vi "Main.vi"() -> ()   [LabVIEW 2013]
uses:
  Controls/Setup - Part Details - Item Details.ctl
  Controls/Combo Box.ctl
  Controls/Execute - Info.ctl
  Controls/Enum - SRTRS State.ctl
  Controls/DB - Refnums.ctl
  Controls/Report Files Cluster.ctl
  Controls/DB - Refnums II.ctl
  Controls/Transaction Cluster.ctl
  Controls/Report List Cluster.ctl
  Controls/DB - Logon Info.ctl
  Controls/DB - Logon Extra Info.ctl
  Controls/ET3500 Program Status.ctl
  <vilib>/Utility/miscctls.llb/LVRowAndColumnUnsignedTypeDef.ctl
  <vilib>/Utility/miscctls.llb/LVPointTypeDef.ctl
  Controls/Execute - Color Init.ctl
  <vilib>/Utility/miscctls.llb/LVRowAndColumnTypeDef.ctl
  Controls/Enum - Tabs.ctl
  Controls/DB - Setup Item Enum.ctl
  Controls/Msgbox Timer Cluster.ctl
  Controls/cRIO RW Enum.ctl
  Controls/DB - Execute Transaction Enum.ctl
  Controls/DB - [TransactionResult] Enum.ctl
  Controls/DB - CMS Execute Active Process.ctl
  Controls/DB - [Execute].[ActiveProcess] Enum.ctl
  Controls/DB - Execute ReportList Enum.ctl
  Controls/DB - [TransactionNo],[OrderNo].ctl
  Controls/DB - Master Data OutputSet SQL.ctl
  Controls/DB - OpenClose.ctl
  Controls/Report Additional Details Cluster.ctl
  Controls/Message Code - Enum.ctl
  <vilib>/event_ctls.llb/eventvkey.ctl
  Controls/DB - Master Data Material Enum.ctl
  Controls/DB - Master Data Procedure Enum.ctl
  <vilib>/Utility/miscctls.llb/LVSelectionTypeDef.ctl
  Controls/DB - [Config].[Parameters].[ParameterId] Values.ctl
  Controls/DB - [Config].[GeneralSetting].[SystemId] Values.ctl
  Controls/Key Enum.ctl
  Controls/Global SRTRS.vi
  <vilib>/Utility/config.llb/Write Key (String).vi
  <vilib>/nisyscfg/Close (System).vi
  <vilib>/addons/database/Connection.llb/DB Tools Open Connec (String).vi
  <vilib>/Utility/config.llb/Write Key (Boolean).vi
  <vilib>/express/express shared/transition.llb/Dynamic To Waveform Array.vi
  <vilib>/express/express signal manip/GetorSetDDTAttributes/Set DDT Attributes/SetT0.vi
  <vilib>/express/express shared/transition.llb/Waveform Array To Dynamic.vi
  <vilib>/Waveform/WDTOps.llb/WDT Get Waveform Subset DBL.vi
  <vilib>/express/express signal manip/GetorSetDDTAttributes/Set DDT Attributes/Set DDT Properties.xnode
  <vilib>/Utility/config.llb/NI_LVConfig.lvlib
  <vilib>/nisyscfg/nisyscfg.lvlib
  <vilib>/FTP/NI_FTP.lvlib
  <vilib>/addons/database/NI_Database_API.lvlib
  SubVIs/tool_Unicode_Convert ASCII to Unicode (Scalar).vi
panel:
  out "[Remarks] +[ShortDescription] Debug":string caption="[Remarks] +[ShortDescription]"
  out "Time To Log Off":dbl(slide)=599.8004469871521 scale=0.0..600.0
  in  "Tab Header":enum32{"Header"}(tab)
  out "Plant and Furnace Name":string="One Subsea Johor, SRSB-A1, Administrator"
  in  "Close":bool
  out "ApplicationName":string caption="[LogoName]"
  out "LogoName":picture
  in  "Debug Close":bool
  in  "Setup Load Debug":bool
  in  "Tab Footer":enum32{"Footer"}(tab)
  out "date/time string":string="Nov 22, 2014  15:42:28"
  out "[Remarks] +[ShortDescription]":string
  in  "Tab Body":T1(tab)
  in  "Search Setup":bool caption="Setup Save"
  in  "Setup New":bool
  in  "Setup Edit":bool=TRUE
  out "Transaction No":string caption="Transaction No."
  in  "Tab Setup":enum32{"Part Details", "Furnace Settings"}(tab) caption="Setup"
  in  "SAPMaterial Description (Long) Setup Tab":bool
  in  "SAPProduction Long Text":bool
  in  "Channel Mapping":T2 caption="Channels Mapping"
  in  "Item Details":T3={"Order No."="", "Oper. No."="", "Qty."=1, "NCR No."="", "NCR Boolean"=FALSE, "Customer No."="", "Customer Name"="", "Project"="", "Sales Order"="", "Item No."="", "Material"="", "Revision"="", "Material Description"="", "Serial No."="", "UnitOfQty"=""} {"Qty." min=1 max=99}
  in  "Part Details Delete":bool
  in  "Part Details Add":bool
  in  "Notes":string
  in  "No.":i32=1 caption="Item Number" min=1 max=100
  out "Setup Thermocouple Location":picture caption="Thermocouples Position: Outline"
  in  "Part Details":i32(listbox)=-1
  in  "Plot":T4
  in  "FHS Ramp Rate Units":string="°C"
  in  "Ramp Rate (Brackets)":string caption="(       / Hour )"
  in  "Target Temperature (Brackets)":string caption="(        )"
  in  "Hold Time (Brackets)":string caption="(HH:MM)"
  in  "Results Output":cluster{"Output Set":T5, "Description":string}={"Output Set"="001", "Description"="Output Set 1"}
  in  "Extra Rev":string caption="Rev."
  in  "Extra WPS":string caption="WPS"
  in  "Read ET3500 Program":bool
  in  "FHS Target Temp Units":string="°C"
  in  "MCListBox AWPS Remove Button":bool
  in  "MCListBox AWPS Add Button":bool
  out "Equipment Details":i32(listbox)=-1
  out "Furnace Details":T6={"Furnace Serial No"="A1234A1", "Last Calibration Date"="2012-11-22", "Next Calibration Due Date"="2014-11-22"}
  in  "Additional WPS/Ref":T7 caption="Additional WPS"
  in  "WPS Details Setup":T8={"WPS/Ref"="", "Rev"="", "Hold Temperature"="", "WPS Details Temperature Units"="°C", "Hold Time (HH:MM)"="", "Inactive"=FALSE} caption="WPS Details"
  in  "MCListBox AWPS":i32(listbox)=-1 caption="Additional WPS/Ref MCListBox"
  in  "MCListBox FHS Setup Add Button":bool
  in  "MCListBox FHS Setup Remove Button":bool
  in  "MCListBox FHS Setup":i32(listbox)=-1 caption="Furnace Heating Sequence"
  in  "Setup Save":bool
  out "TransactionRunNo":string caption="Run No."
  in  "Copy New":bool caption="Setup Save"
  in  "Transaction Details":bool
  in  "System Status [CaptionOnly] 2":string caption="System Status"
  in  "Process Status [CaptionOnly]":string caption="Process Status"
  out "% Hold. Time Completed (Num)":i32 format="%d%%"
  out "Overall Status":bool
  out "Sequence Status":string caption="Sequence"
  in  "Parameter":bool
  out "ET3504 Status":string="Program [33]. Segment [End].Program Status [Not Running]. ET3500 Simulate Mode." caption="Furnance"
  out "Info.":T9={"Ref WPS"="", "Hold. Temp."="", "Info. Temperature Units"="°C", "Variant Allowed (Hold Temp)"=5.0, "Info. Temperature Units 2"="°C", "Variant Allowed (Hold Temp)"=FALSE, "Hold. Time (hour:minute)"="", "Variant Allowed (Hold Time)"=30.0, "Variant Allowed (Hold Time)"=FALSE, "WPS"=""} {"Variant Allowed (Hold Temp)" format="%.1f"}
  out "Hold Time Completed":bool
  out "Process Completed":bool
  out "% Hold. Time Completed":dbl(slide) scale=0.0..100.0
  out "Transaction No (Execute)":string caption="Transaction No."
  out "Key Values":T10={"Recording Duration"=0.0, "Remaining Hold Time"=0.0, "Current Temp"=25.108964136983314, "Key Values Temperature Units"="°C"} {"Current Temp" format="%#_4f"; "Remaining Hold Time" format="%<%H:%M>t"; "Recording Duration" format="%<%H:%M:%S>t"}
  out "Chart":dynamicdata(graph)
  in  "Recipe Start":bool
  in  "Recipe Stop":bool
  out "cRIO Status":string="DAQ Waiting to Start. cRIO Simulate Mode." caption="Data Logger"
  out "TransactionRunNo (Execute)":string caption="Run No."
  in  "Probe Number [CaptionOnly]":string caption="Probe Number"
  in  "Create Report [CaptionOnly]":string caption="Create Report"
  in  "Retrieve Raw Data [CaptionOnly]":string caption="Retrieve Raw Data"
  in  "Display Report [CaptionOnly]":string caption="Display Report"
  in  "cRIO FTP Copy":bool caption="Report Execute Search"
  in  "FTP File List":i32(listbox)=-1
  in  "cRIO  Search":bool caption="Report Execute Search"
  in  "FTP Month":i16=11 caption="Month" min=1 max=12 format="%02d"
  in  "FTP Year":i16=2014 caption="Year" min=2013 max=2099
  in  "Report Open":bool caption="Report Execute Search"
  in  "Report List":i32(listbox)=-1 caption="List"
  in  "Report Generate":bool
  in  "Raw Data File (Report Tab)":path caption="Raw Data File"
  in  "Report Selection":T11={"Date Start"=timestamp(3498882134.864412 s since 1904-01-01), "Date End"=timestamp(3499486934.864412 s since 1904-01-01), "Selection Transaction No"="", "Selection Order No"="", "Report Execute Search "=FALSE} caption="Selection" {"Date End" format="%<%Y/%m/%d>T"; "Date Start" format="%<%Y/%m/%d>T"}
  in  "Master Data Tab":enum32{"Material", "WPS", "Layout"}(tab) caption="Tab Master Data"
  in  "Material Reference [CaptionOnly]":string caption="Reference"
  in  "Master Data Ref Material":string(combo) caption="Material"
  in  "Material Details [CaptionOnly]":string caption="Material Details"
  in  "SAPMaterial Description (Long) Master Data Tab":bool
  in  "Material Paste":bool caption="Material Browse"
  in  "Material Copy":bool caption="Material Browse"
  in  "Material":T12 caption="Header"
  in  "Material New":bool
  in  "Material Browse":bool
  in  "Material Save":bool caption="Material Add"
  out "Master Data Thermocouple Location":picture caption="Thermocouples Position: Outline"
  in  "WPS Details [CaptionOnly]":string caption="WPS Details"
  in  "MasterData FHS Target Temp Units":string="°C"
  in  "MasterData FHS Ramp Rate Temp Units":string="°C"
  in  "WPS Details Master Data":T13={"Master Data WPS/Ref"="", "Master Data Rev"="", "Master Data Hold Temperature"="", "Master Data Temperature Units"="°C", "Master Data Hold Time (HH:MM)"="", "Inactive"=FALSE} caption="Header"
  in  "MCListBox FHS Master Data":i32(listbox)=-1 caption="Furnance Heating Sequence"
  in  "Master Data New":bool
  in  "Master Data Save":bool
  in  "MCListBox FHS Master Data Remove Button":bool
  in  "MCListBox FHS Master Data Add Button":bool
  in  "Output Details [CaptionOnly]":string caption="Output Details"
  in  "Admin (User/Equipment) Tab":enum32{"User", "Equipment"}(tab)
  in  "User Details [CaptionOnly]":string caption="User Details"
  in  "Equipment Details [CaptionOnly]":string caption="Equipment Details"
  in  "System Status [CaptionOnly]":string caption="System Status"
  out "Material Image File":errorcluster
  out "Statistics":errorcluster
  out "Chart":errorcluster
  out "Property Node Error":errorcluster
  in  "Mytab":T14(tab)
  in  "MasterData\\Language":path=path "c:/temp/SRTRS4070/MasterData/Language"
  in  "MasterData\\Layout":path=path "c:/temp/SRTRS4070/MasterData/Layout"
  in  "Setup":path=path "c:/temp/SRTRS4070/Setup"
  in  "MasterData\\WPS":path=path "c:/temp/SRTRS4070/MasterData/WPS" caption="Master Data WPS"
  in  "MasterData\\JPG":path=path "c:/temp/SRTRS4070/MasterData/JPG"
  in  "Data":path=path "c:/temp/SRTRS4070/Data" caption="Folder Data"
  in  "Excel":path=path "c:/temp/SRTRS4070/Excel" caption="Folder Excel"
  in  "Logs":path=path "c:/temp/SRTRS4070/Logs"
  in  "Reports":path=path "c:/temp/SRTRS4070/Reports" caption="Folder Report"
  in  "Temp_Host":path=path "c:/temp/SRTRS4070_Host/Temp_Host"
  in  "Data_Host":path=path "c:/temp/SRTRS4070_Host/Data_Host" caption="Folder Data"
  in  "Logs_Host":path=path "c:/temp/SRTRS4070_Host/Logs_Host"
  in  "Dummy Load":bool caption="Show Debug Tab"
  out "Update English Captions":bool
  out "Display Reference Chart":bool=TRUE
  out "Settings Load Sequence":i32[](array[numeric])=[0, 1, 2]
  out "Date Format (UserDefined)":string="%Y-%m-%d"
  out "Starting Number for Transaction number":i32=1000000001
  out "Display Start Stop Marker":bool=TRUE
  out "ini File Error":errorcluster
  out "Log Off Timer (s)":i32=600
  out "Chart Separation by Order#":bool=TRUE
  out "Lite Version":bool
  out "stp file Error Out":errorcluster
  out "Furnace Number":string="03"
  out "Running Number":i32=829
  out "Show Debug TAB":bool=TRUE caption="Show Debug Tab"
  out "Show LabVIEW Error":bool
  out "Application:Name":string="LabVIEW.exe"
  out "Metrics:Code Size":u32=1762288 format="%#.3p"
  out "MCListBox Ref":refnum<vi>[](array[refnum])
  in  "CellBG ColHdrs":u32(colorbox)=11776947
  in  "CellBG Unused Cells":u32(colorbox)=16777238
  in  "CellBG New Cells":u32(colorbox)=16777225
  out "Latest stp file":path=path "c:/temp/SRTRS4070/Setup/2014/11/0090300828_20141120_120827.stp"
  out "LabVIEW Directory Path":path=path "C:/Program Files (x86)/National Instruments/LabVIEW 2013"
  out "All Calibration Date Valid":bool
  out "Calibration Date OK":bool[](array[boolean])
  out "User":string="admin"
  in  "Edit WPS in Setup":bool
  out "Final Logoff Timer (s)":i32=600
  out "Temperature Units":refnum<vi>[](array[refnum])
  out "SRTRS4070 Host Folder":string="c:\\temp\\SRTRS4070_Host"
  out "SRTRS4070 Folder (Server Folder)":string="c:\\temp\\SRTRS4070"
  out "LogoName":errorcluster
  out "Current VI's path":path=path "C:/Users/CK/workspace/LabVIEW/Stress Relief Temperature Recording/VIs/Main.vi"
  out "Application Directory":path=path "C:/Users/CK/workspace/LabVIEW/Stress Relief Temperature Recording"
  out "[TimeZone]":string="+8"
  out "Enable Central Monitoring":bool=TRUE
  out "File Version":string="ver. 13.0f1"
  out "Plant and Furnace Name (B4 Logon)":string="ver. 13" caption="Plant and Furnace Name"
  out "[LogoFile]":string="C:\\Temp\\SRTRS4070_Host\\Temp_Host\\OneSubseaLogo.jpg"
  out "Caption Error Out":errorcluster
  out "Enable AMS Update":bool=TRUE
  out "Equipment ID Notice Due List":string
  out "Equipment Details Complete":bool caption="Output Set Complete"
  in  "Setup New Toggle":bool caption="Report Generate Procedure"
  in  "Search [OrderNo] Toggle":bool caption="Report Generate Procedure"
  out "From Search Button":bool caption="Report Generate Procedure"
  out "Channel to Probe Mapping":cluster{"Channel to Probe Mapping":string}={"Channel to Probe Mapping"="1,2,3,4,5,6,7,8,9,10,11,12,13,14,15,16"}
  out "Probe List":i32[](array[numeric])
  out "Probe List Valid":bool
  out "cRIO Channel List":i32[](array[numeric])
  out "Empty String in Mandatory Field":bool
  out "WPS Details Complete":bool
  out "FHS Last Row":i32
  out "[Setup].[Item] COLUMN_NAME":string[](array[string])=["TransactionNo", "ItemNo", "OrderNo", "OperationNo", "Qty", "UnitOfQty", "NCRIndicator", "NCRNo", "CustomerID", "Customer", "Project", "SalesOrderNo", "SalesOrderItemNo", "MaterialNo", "MaterialDesc", "MaterialRev", "SerialNos", "Notes", "TC01", "TC02", "TC03", "TC04", "TC05", "TC06", "TC07", "TC08", "TC09", "TC10", "TC01Plot", "TC02Plot", "TC03Plot", "TC04Plot", "TC05Plot", "TC06Plot", "TC07Plot", "TC08Plot", "TC09Plot", "TC10Plot", "Inactive"]
  out "[Setup].[Item] DATA_TYPE":string[](array[string])=["int", "int", "nvarchar", "nvarchar", "int", "nvarchar", "nvarchar", "nvarchar", "nvarchar", "nvarchar", "nvarchar", "nvarchar", "nvarchar", "nvarchar", "nvarchar", "nvarchar", "nvarchar", "nvarchar", "nvarchar", "nvarchar", "nvarchar", "nvarchar", "nvarchar", "nvarchar", "nvarchar", "nvarchar", "nvarchar", "nvarchar", "nvarchar", "nvarchar", "nvarchar", "nvarchar", "nvarchar", "nvarchar", "nvarchar", "nvarchar", "nvarchar", "nvarchar", "bit"]
  out "[Setup].[Item] PRECISION":string[](array[string])=["10", "10", "10", "5", "10", "5", "50", "20", "10", "30", "30", "10", "6", "20", "60", "3", "255", "255", "2", "2", "2", "2", "2", "2", "2", "2", "2", "2", "1", "1", "1", "1", "1", "1", "1", "1", "1", "1", "1"]
  out "[IsMandatory]":string[](array[string])=["0", "0", "0", "0", "-1", "0", "-1", "0", "0", "-1", "", "", "0", "0"]
  out "[IsMandatory]\nLabel.Text":string[](array[string])=["Customer No.", "Project", "Material"]
  in  "Search Setup Toggle":bool caption="Report Generate Procedure"
  out "Revision Toggle":string caption="Report Generate Procedure"
  out "Part Details Complete":bool caption="WPS Details Complete"
  out "Output Set Details Complete":bool caption="Output Set Complete"
  out "FHS Hold Details Complete":bool caption="WPS Details Complete"
  out "Equipment ID Due List":string
  out "TCxxPlots 2":string[][](array[string])
  out "TCxxPlots":bool
  out "<current hold time> ON Failing Hold Time Variance":string
  in  "Simulate Hold Time Inc (s)":dbl=2400.0
  out "Toggle ET3500 Error":string
  in  "Simulate Hold Temp Inc":dbl=20.0
  out "Final Target Temperature":cluster{"Final Target Temperature":string}
  in  "Parameter Buffer":T15
  out "Parameter (End Dwell Time)":timestamp
  out "Parameter (Start Dwell Time)":timestamp
  out "ET3500 Error":errorcluster
  in  "Simulate ET3500":bool=TRUE
  out "Parameter Cluster (Scaled)":T16={"ProgramNumber"=1, "CurProg"=33, "CurSeg"=1, "ProgStatus"=1, "ProgTimeLeft (min)"=0.0, "PVIn (DegC)"=25.108964136983314, "SPIn (s)"=0.0, "SegTimeLeft (min)"=9.0}
  in  "Simulate ET3500 Error":bool
  in  "Final Target Temp Offset":i32
  in  "Stop On Final Target Temperature":bool=TRUE
  out "Final Target + Offset\n(Updated Only when active)":i32
  out "Seq-Seg Info":T17
  out "Uploaded to ET":bool caption="ET Program Downloaded"
  in  "Simulate Hold Temp Inc":bool
  in  "Simulate Hold Time Inc":bool
  out "Hold Time %":string
  out "<current temperature> ON Failing Hold Temp Variance":string
  out "cRIO Time Sync Schedule":i32=700 caption="cRIO Time Sync Tolerance"
  in  "Simulate cRIO No Data":bool
  out "cRIO DAQ Started":bool
  out "cRIO Error":errorcluster
  out "cRIO Cycle Count":i32
  out "cRIO shared variable RT Library":string="ni.var.psp://192.168.1.50/RT Library"
  out "VISA resource name RS232":string="visa://192.168.1.50/ASRL1::INSTR"
  out "Samples/ch Count":i32
  out "cRIO COM Port":string="visa://192.168.1.50/ASRL1::INSTR"
  out "Host COM Port":string="COM3"
  out "cRIO IP":string="192.168.1.50"
  out "cRIO Folder":string="/c/ni-rt/LabVIEW Data/SRTRS4070"
  in  "Simulate cRIO":bool=TRUE caption="Simulate cRIO Data"
  in  "Use Host COM Port":bool
  out "cRIO Data Retention":i32=3
  out "cRIO Timestamp":timestamp
  in  "Simulate cRIO Comm Error":bool
  in  "Simulate cRIO Started":bool
  out "1st TC":dbl
  out "Data Path Name (cRIO SV)":string
  out "Files in cRIO":string[](array[string])
  out "cRIO File IO Status (updated at File creation only)":bool[](array[boolean])
  out "Check DAQ Started Loop Count":i32
  out "Day cRIO Time is SET":string
  out "SV and ini Data File Name Match. (Recovery)":bool
  out "Simulated TimeStamp":timestamp
  out "cRIO Time Sync Tolerance":i32=60
  out "Source File Path (on RT Target)":string
  out "Destination Folder (on Local Host)":path
  out "Destination File Path (on local host)":path
  out "cRIO FTP Module (Error Out)":errorcluster
  out "Data File Error":errorcluster
  out "Logged File Ref":refnum<file>
  out "Time to next sample (s)":dbl
  out "Host Sampling Interval (s)":dbl=1.0
  in  "Time Target (s)":dbl format="%#_13g"
  out "Raw Data File":string
  out "[StartRecordTime]":string
  out "RecoveryFlag":bool
  out "Recovered Data Size":i32[](array[numeric])
  out "Calculate Parameters from raw Data":string[](array[string])
  out "Variant Allowed (Hold Time) (raw Data)":bool
  out "Variant Allowed (Hold Temp) (raw Data)":bool
  out "|Max - Hold Temp|":dbl
  out "|Min - Hold Temp|":dbl
  out "|Hold - Hold Time|":dbl
  in  "Sort Order":bool caption="Include MetaData"
  in  "Include MetaData":bool=TRUE
  out "ReportList Cluster":T18
  out "Transaction (Report Buffer)":T19
  out "List Of Files From Selected Reports":string[](array[string])
  out "YYYYmm":string
  out "Details From .stp and Parameters":string[](array[string])
  out "Order No":string[](array[string])
  in  "Report.Create.PDF":bool=TRUE caption="Create PDF file at end of Recipe"
  in  "Report.Create.Excel":bool=TRUE caption="Create EXCEL file at end of Recipe"
  out "No Of Orders":i32
  out "Report Files Cluster":T20
  in  "Report Generate Toggle":bool=TRUE caption="Report Generate Procedure"
  out "Logon (Report Buffer)":T21
  out "Msgbox":errorcluster
  out "Ascending":bool
  out "Template File":path
  out "Layout ID":string
  out "Manual Stop":bool caption="Manual Stop Flag"
  out "Stop Log off Event Structure":bool=TRUE
  in  "------------------------------------        Setup TAB      ------------------------------------":string caption="------------------------------------        Setup Tab     ------------------------------------"
  in  "---------------------------------       Master Data (Material)      -----------------------------":string
  out "Temp Array":string[](array[string])
  out "Time has Elapsed":bool
  out "Quit Flag":bool=TRUE
  out "Recipe Start Flag":bool
  out "Recipe Stop Flag":bool
  out "WPS Details Master Data: Mouse Down":u32 caption="Time"
  out "Process t0":timestamp
  out "MasterData Image File Path":path caption="MasterDate Image File Path"
  in  "------------------------------------        Master Data       -----------------------------------":string
  in  "------------------------------------        MCListBox       ------------------------------------":string
  in  "-------------------------------             Report TAB        ------------------------------------":string caption="------------------------------------             Report          ------------------------------------"
  in  "------------------------------------        Part Details       ------------------------------------":string
  out "StateMachine for Main Process":T22=enum."QUIT" caption="Enum"
  out "Show Scrollbars":bool=TRUE
  out "WPS Details Master Data: Value Change":u32
  out "% Hold Flashing FLAG":bool caption="Time has Elapsed"
  in  "Master Data Delete":bool
  in  "Material Delete":bool
  in  "------------------------------------        Execute TAB      ------------------------------------":string caption="------------------------------------        Setup Tab     ------------------------------------"
  in  "------------------------------------        Simulate TAB      ------------------------------------":string caption="------------------------------------        Setup Tab     ------------------------------------"
  in  "Copy Setup":bool caption="Setup Save"
  in  "Paste Setup":bool caption="Setup Save"
  in  "cRIO Set Time":bool
  out "No. of Items":i32
  in  "Reset Log off Display Timer":bool caption="Reset"
  out "MHandler":errorcluster caption="Message Handler Error"
  in  "DB - Active Process":bool=TRUE
  in  "DB - Message":bool=TRUE
  in  "DB - Report":bool=TRUE
  in  "DB - Logon":bool=TRUE
  in  "DB - Transaction":bool=TRUE
  in  "DB - Setup Item (Part Details)":bool=TRUE
  in  "DB - Master Data Load":bool=TRUE
  in  "DB - Master Data Save":bool=TRUE
  out "DB":errorcluster
  out "DB Refnums":T23
  out "[Config].[Parameter]":string[][](array[string])=[["AllowWpsEdit", "0"], ["ChartSeparation", "1"], ["DataLogInterval", "1"], ["DateFormat", "%Y-%m-%d"], ["DisplayRefChart", "1"], ["EnableCmsUpdate", "1"], ["NotifySeverity", "5,6,8,9"], ["PermittedTempDiff", "5"], ["PermittedTimeDiff", "30"], ["StartStopMarker", "1"]]
  out "DB Refnums II":T24
  out "[Config].[GeneralSetting]":string[][](array[string])=[["GenericSystemId", "ALL"], ["ScreenLockTimer", "600"], ["TimeSyncSchedule", "07:00"], ["TimeSyncTolerance", "60"], ["TransactStartNo", "1000000001"]]
  out "Layout UI":refnum<vi>
  out "SubPanel":errorcluster
  out "Logon OK":bool=TRUE
  in  "[RawDataReport]":bool=TRUE
  in  "[TabUserAccess]":bool[](array[boolean])=[TRUE, TRUE, TRUE, TRUE, TRUE, TRUE, TRUE, TRUE, TRUE, TRUE, TRUE, TRUE, TRUE, TRUE, TRUE, TRUE, TRUE, TRUE, TRUE, TRUE]
  in  "Logon Extra":T25={"Plant Name"="One Subsea Johor", "UserName"="Administrator", "Hostname [ClientName]"="CK_HP-Envy", "IsUnicode"=FALSE}
  in  "Logon":T21={"PlantID"="4070", "SystemID"="SRSB-A1", "UserID"="admin", "DomainID"="Local", "LanguageID"="EN", "StationID"="F001"}
  in  "Application":string="SRTRS"
  out "Admin Equipment UI":refnum<vi>
  out "Config UI":refnum<vi>
  in  "Stop":bool
  out "UI Event":errorcluster={"status"=TRUE, "code"=1026, "source"="Close Reference in Main.vi"}
  out "Execution:State":T26(ring)=enum."Idle"
  out "Front Panel Window:State":T27(ring)=enum."Closed"
  out "Admin User UI":refnum<vi>
  out "Logon UI":refnum<vi>
  in  "WPS Details Buffer":T28={"WPS/Ref"="", "Rev"="", "Hold Temperature"="", "WPS Details Temperature Units"="°C", "Hold Time (HH:MM)"="", "Extra WPS"="", "Extra Rev"=""}
  in  "Material Buffer":T12 caption="Header"
  out "WPS Details Buffer (DB)":T13
  out "Copy/Paste DB Ref Nums":errorcluster
  out "[OutputSetId],[Description]":string[][](array[string])
  out "MessageQ":string="000012\t20141122_154228\tQUIT\n000011\t20141122_154228\t<APP><W 113> {Debug CLOSE}\n000010\t20141122_154217\t[Config UI] UI Load OK.\n000009\t20141122_154217\t[Admin User UI] UI Load OK.\n000008\t20141122_154201\t<cRIO><I 402> <NoD> Simulate cRIO Set Time. <NoD>\n000007\t20141122_154201\t<cRIO><I 400> {Ready to Start} Time Difference is 2147483647 seconds. cRIO DAQ NOT Started. cRIO Comm GOOD.  <NoD>\n000006\t20141122_154200\t<APP><I 110> \n000005\t20141122_154200\t<DB><I 302> cRIO IP = 192.168.1.50 [ChannelMapping] = 1,2,3,4,5,6,7,8,9,10,11,12,13,14,15,16 <NoD>\n000004\t20141122_154200\t<APP><I 110> [UserID] = admin, [UserName] =  Administrator, [PlantId] =  4070, [SystemId] =  SRSB-A1 <NoD>\n000003\t20141122_154158\t[Logon UI] UI Load OK.\n000002\t20141122_154157\t\"c:\\temp\\SRTRS4070_Host\\Logs_Host\\2014\\11\\20141122_154157.log\" Event File Created.\n000001\t20141122_154157\tReady to Start.\n000000\t20141122_154157\t<APP><I 100> {Initialization}<APP><I 100> SRTRS Initialize OK.\"C:\\Users\\CK\\workspace\\LabVIEW\\Stress Relief Temperature Recording\\SRTRS.ini\" is Loaded. 52 out of 52 Keys are FOUND.  Code Size = 1762288. <NoD>\n\n\n\n\n\n\n\r\n"
  out "State Machine Error Out":errorcluster
  out "Event File Error":errorcluster
  out "MessageQ Error":errorcluster
  out "System Status":errorcluster
  # "Thermocouple"
  # "Probe No."
  # "(hh:mm:ss)"
  # "(hh:mm)"
  # "Min"
  # "to"
  # "Date"
  # "OR"
  # "(      )"
  # "(HH:MM)"
  # "(     /Hour )"
  # "Logon"
  # "From [Config].[Parameter] / [Config].[Setting]"
  # "(only updated when a Shared Variable is Read)"
  # "FTP Copy (RETR)"
  # "c:\n\nu:"
  # "HoldTimeMaxTemp\nHoldTimeMaxTempTime\nHoldTimeMinTemp\nHoldTimeMinTempTime\nTempDiffDuringHold\n--------------------------\nMaxRecordedTemp\nMaxRecordedTempTime\nMinRecordedTemp\nMinRecordedTempTime\nTempDiffDuringHold"
  # "Not in use anymore"
  # "Initialized during Initialization Sequence"
  # "Updated after Logon"
  # "Min"
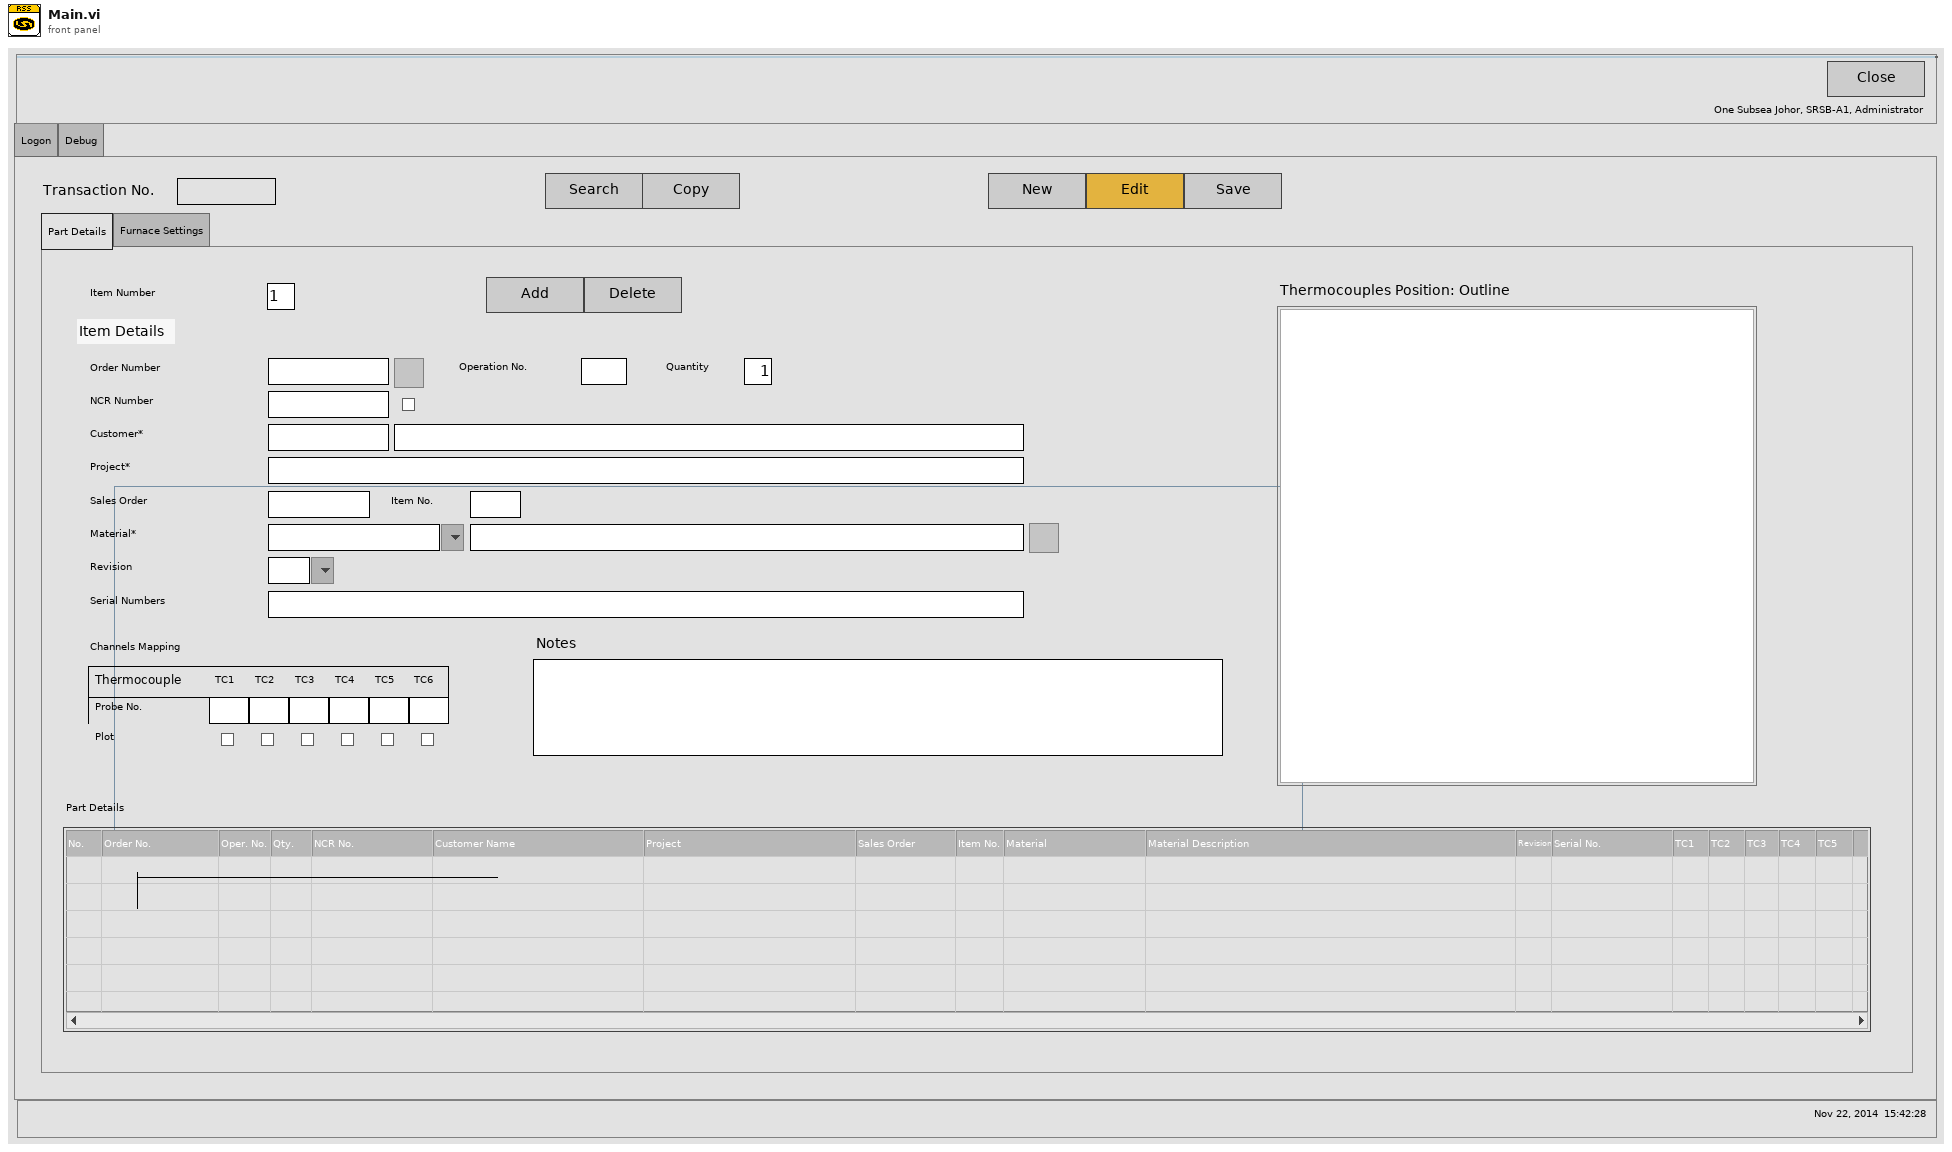
[diagram p1: front panel]
types:
  T1 = enum32{"Setup", "Execute", "Report", "Master Data", "Admin", "Config", "Logon", "Debug"}
  T2 = cluster{"TC1":string, "TC2":string, "TC3":string, "TC4":string, "TC5":string, "TC6":string}
  T3 = typedef "Setup - Part Details - Item Details.ctl" = cluster{"Order No.":string, "Oper. No.":string, "Qty.":i32, "NCR No.":string, "NCR Boolean":bool, "Customer No.":string, "Customer Name":string, "Project":string, "Sales Order":string, "Item No.":string, "Material":string, "Revision":string, "Material Description":string, "Serial No.":string, "UnitOfQty":string}
  T4 = cluster{"TC01Plot":bool, "TC02Plot":bool, "TC03Plot":bool, "TC04Plot":bool, "TC05Plot":bool, "TC06Plot":bool}
  T5 = typedef "Combo Box.ctl" = string
  T6 = cluster{"Furnace Serial No":string, "Last Calibration Date":string, "Next Calibration Due Date":string}
  T7 = cluster{"Additional WPS/Ref":T5, "Additional Rev":T5}
  T8 = cluster{"WPS/Ref":T5, "Rev":T5, "Hold Temperature":string, "WPS Details Temperature Units":string, "Hold Time (HH:MM)":string, "Inactive":bool}
  T9 = typedef "Execute - Info.ctl" = cluster{"Ref WPS":string, "Hold. Temp.":string, "Info. Temperature Units":string, "Variant Allowed (Hold Temp)":dbl, "Info. Temperature Units 2":string, "Variant Allowed (Hold Temp)":bool, "Hold. Time (hour:minute)":string, "Variant Allowed (Hold Time)":dbl, "Variant Allowed (Hold Time)":bool, "WPS":string}
  T10 = cluster{"Recording Duration":dbl, "Remaining Hold Time":dbl, "Current Temp":dbl, "Key Values Temperature Units":string}
  T11 = cluster{"Date Start":timestamp, "Date End":timestamp, "Selection Transaction No":T5, "Selection Order No":T5, "Report Execute Search ":bool}
  T12 = cluster{"Master Data Material":string, "Master Data Rev":string, "Master Data Material Description":string, "Inactive":bool}
  T13 = cluster{"Master Data WPS/Ref":T5, "Master Data Rev":T5, "Master Data Hold Temperature":string, "Master Data Temperature Units":string, "Master Data Hold Time (HH:MM)":string, "Inactive":bool}
  T14 = enum32{"Paths", "Host Paths", "Settings", "Part Details Add/Edit", "ET3500", "cRIO", "Data File", "Report", "Others", "DB", "SubPanel", "Buffers"}
  T15 = cluster{"Start Holding Time and Date":string, "End Holding Time and Date":string, "Start Holding Temperature":string, "End Holding Temperature":string}
  T16 = cluster{"ProgramNumber":i16, "CurProg":i16, "CurSeg":i16, "ProgStatus":i16, "ProgTimeLeft (min)":dbl, "PVIn (DegC)":dbl, "SPIn (s)":dbl, "SegTimeLeft (min)":dbl}
  T17 = cluster{"Main Hold Sequence#":i32, "End Segment#":i32}
  T18 = typedef "Report List Cluster.ctl" = cluster{"[LayoutId]":string, "[OrderNo]":string, "[ReportRunNo]":string, "[NoOfOrders]":string, "[ReportFilePath]":string, "[ReportFileName]":string, "[RawDataSourcePath]":string, "[RawDataSourceFileName]":string, "[IsManual]":string}
  T19 = typedef "Transaction Cluster.ctl" = cluster{"TransactionNo":string, "TransactionRunNo":string}
  T20 = typedef "Report Files Cluster.ctl" = cluster{"Reports":path, "MasterData\\JPG":path, "Excel Template":path, "Report Filename":path, "Raw Data File":path, "Temp_Host":path}
  T21 = typedef "DB - Logon Info.ctl" = cluster{"PlantID":string, "SystemID":string, "UserID":string, "DomainID":string, "LanguageID":string, "StationID":string}
  T22 = typedef "Enum - SRTRS State.ctl" = enum16{"READY TO START", "START Recipe", "START Recovery", "BEGIN Process", "RUNNING Process", "END Process", "Spare Enum", "END Recipe", "ERROR Handling", "QUIT"}
  T23 = typedef "DB - Refnums.ctl" = cluster{"Item Details":refnum<vi>, "WPS Details":refnum<vi>, "WPS (Extra)":refnum<vi>, "Rev (Extra) ":refnum<vi>, "FHS MCListbox":refnum<vi>, "Additional WPS/Ref MCListBox":refnum<vi>, "Notes":refnum<vi>, "Part Details (MClistBox)":refnum<vi>, "Result Output":refnum<vi>}
  T24 = typedef "DB - Refnums II.ctl" = cluster{"Furnace Details":refnum<vi>, "CompactRIO Module Details":refnum<vi>, "Info. (Execute Tab)":refnum<vi>}
  T25 = typedef "DB - Logon Extra Info.ctl" = cluster{"Plant Name":string, "UserName":string, "Hostname [ClientName]":string, "IsUnicode":bool}
  T26 = enum32{"Bad", "Idle", "Run top level", "Running"}
  T27 = enum32{"Invalid", "Standard", "Closed", "Hidden", "Minimized", "Maximized"}
  T28 = cluster{"WPS/Ref":T5, "Rev":T5, "Hold Temperature":string, "WPS Details Temperature Units":string, "Hold Time (HH:MM)":string, "Extra WPS":string, "Extra Rev":string}
  T29 = typedef "ET3500 Program Status.ctl" = enum16{"Wait For RUN", "Running", "Stopped"}
  T30 = enum8{"Enabled", "Disabled", "Disabled and Grayed Out"}
  T31 = enum16{"Always On", "Always Off", "Off While Running"}
  T32 = typedef "LVPointTypeDef.ctl" = cluster{"Horizontal":i16, "Vertical":i16}
  T33 = typedef "LVRowAndColumnTypeDef.ctl" = cluster{"Row":i32, "Column":i32}
  T34 = typedef "LVRowAndColumnUnsignedTypeDef.ctl" = cluster{"Row":u32, "Column":u32}
  T35 = enum32{"Page Enabled", "Page Disabled", "Page Disabled & Grayed"}[]
  T36 = typedef "Execute - Color Init.ctl" = cluster{"Color Box":u32, "Color Box 2":u32}[]
  T37 = cluster{"SRTRS4070 Folder":string, "cRIO Folder":string, "cRIO IP":string, "Temperature Units":string, "Furnace Number":string, "Plant and Furnace Name":string, "LogoFile":string, "Software Solution Name":string, "Channel to Probe Mapping":string, "Running Number":string, "Permitted Temperature Difference":string, "Permitted Time Difference":string, "Host COM Port":string, "Host Sampling Interval":string, "cRIO Data Retention":string, "cRIO Time Sync Schedule":string, "cRIO Time Sync Tolerance":string, "Date Format":string, "SRTRS4070 Host Folder":string, "Latest stp File":string, "Log Off Timer":string, "Raw Data File":string, "Layout Details":string}
  T38 = typedef "Connection Information Cluster.ctl" = cluster{"Connection ":string, "Username":string, "Password":string}
  T39 = cluster{"Create EXCEL":bool, "Create PDF":bool, "Simulate cRIO":bool, "Simulate ET3500":bool, "Simulate No DB":bool, "Use Host COM Port":bool, "Show LabVIEW Error":bool, "Show Debug Tab":bool, "Show Scrollbars":bool, "Stop On Final Target Temperature":bool, "Lite Version":bool, "Edit WPS in Setup":bool, "Display Start Stop Marker":bool, "Update English Captions":bool}
  T40 = typedef "imagedata.ctl" = cluster{"image type":i32, "image depth":i32, "image":u8[], "mask":u8[], "colors":u32[], "Rectangle":cluster{"left":i16, "top":i16, "right":i16, "bottom":i16}}
  T41 = enum16{"open", "replace", "create", "open or create", "replace or create", "replace or create with confirmation"}
  T42 = typedef "Enum - Tabs.ctl" = enum32{"Setup", "Execute", "Report", "Master Data", "Admin", "Config", "Logon", "Debug"}
  T43 = typedef "DB - Setup Item Enum.ctl" = enum16{"SELECT [Plant],[OrderNo]", "INSERT [Setup].[Header]", "INSERT [Setup].[Item]", "INSERT [Setup].[ProcedureItem]", "SELECT [TransactionNo]", "SELECT [TransactionNo], others", "SELECT [OrderNo]", "SELECT [OrderNo], others", "SELECT h.[TransactionNo], i.[OrderNo]", "SELECT [Setup].[ProcedureItem]", "SELECT [EquipmentxId]"}
  T44 = typedef "Msgbox Timer Cluster.ctl" = cluster{"Show":bool, "Priority":i32, "Message":string, "seconds":i32}
  T45 = typedef "cRIO RW Enum.ctl" = enum16{"Write", "Read", "Write Others"}
  T46 = enum16{"Blank Cells Only", "Exisiting and Blank Cells"}
  T47 = typedef "DB - Execute Transaction Enum.ctl" = enum16{"INSERT INTO [Header]", "INSERT INTO [TransactionResult]", "INSERT INTO [ProcedureItem]", "INSERT/UPDATE [Execute].[Active]", "SELECT [Execute].[Active]", "UPDATE [TransactionResult]", "UPDATE FILESTREAM", "SELECT [TransactionResult]", "SELECT [TransactionNo],[TransactionRunNo]"}
  T48 = typedef "DB - CMS Execute Active Process.ctl" = enum16{"INSERT INTO [Execute].[ActiveProcess]", "UPDATE [Execute].[ActiveProcess]", "SELECT [Execute].[ActiveProcess]", "UPDATE FILESTREAM", "SELECT FILESTREAM", "Check [IsActive]"}
  T49 = typedef "DB - Execute ReportList Enum.ctl" = enum16{"INSERT INTO [Execute].[TransactionReport]", "UPDATE [Execute].[TransactionReport]", "INSERT INTO [Execute].[ReportList] ", "SELECT [TransactionNo] OR [OrderNo]", "SELECT [TransactionNo],* OR [OrderNo],*", "SELECT [ReportFileName]"}
  T50 = typedef "Report Additional Details Cluster.ctl" = cluster{"[LanguageId]":string, "[ReportRunNo]":string, "[PlantId]":string, "[SystemId]":string}
  T51 = typedef "DB - Master Data OutputSet SQL.ctl" = enum16{"SELECT [OutputSetId]", "SELECT [LayoutFilePath],[LayoutFileName]"}
  T52 = typedef "DB - [TransactionNo],[OrderNo].ctl" = enum16{"h.[TransactionNo]", "h.[ProcedureNo]", "h.[ProcedureRev]", "h.[WPSNo]", "h.[WPSRev]", "h.[HoldTemperature]", "h.[UnitOfTemperature]", "h.[HoldTime]", "h.[AdditionalProcs]", "h.[OutputSetId]", "h.[PermittedTempDiff]", "h.[PermittedTimeDiff]", "j.[Description]", "i.[itemNo]", "i.[OrderNo]", "i.[OperationNo]", "i.[Qty]", "i.[UnitOfQty]", "i.[NCRIndicator]", "i.[NCRNo]", "i.[CustomerID]", "i.[Customer]", "i.[Project]", "i.[SalesOrderNo]", "i.[SalesOrderItemNo]", "i.[MaterialNo]", "i.[MaterialDesc]", "i.[MaterialRev]", "i.[SerialNos]", "i.[Notes]", "i.[TC01]", "i.[TC02]", "i.[TC03]", "i.[TC04]", "i.[TC05]", "i.[TC06]", "i.[TC01Plot]", "i.[TC02Plot]", "i.[TC03Plot]", "i.[TC04Plot]", "i.[TC05Plot]", "i.[TC06Plot]"}
  T53 = typedef "DB - OpenClose.ctl" = cluster{"Open":bool, "Close":bool}
  T54 = typedef "Message Code - Enum.ctl" = enum16{"<APP><I 100>", "<APP><E 101>", "<APP><I 110>", "<APP><W 111>", "<APP><I 112>", "<APP><W 113>", "<APP><I 114>", "<APP><I 115>", "<APP><I 116>", "<APP><W 117>", "<APP><I 120>", "<APP><W 121>", "<APP><E 122>", "<APP><W 130>", "<APP><W 131>", "<APP><W 132>", "<APP><W 133>", "<APP><W 134>", "<DB><I 150>", "<DB><I 151>", "<DB><W 152>", "<APP><I 200>", "<APP><I 201>", "<APP><W 202>", "<APP><E 203>", "<DB><I 300>", "<DB><I 301>", "<DB><W 302>", "<DB><I 305>", "<DB><I 306>", "<DB><W 307>", "<DB><W 310>", "<cRIO><I 400>", "<cRIO><W 401>", "<cRIO><I 402>", "<cRIO><W 403>", "<ET><I 500>", "<ET><W 501>", "<ET><I 600>", "<ET><W 601>", "<ET><E 602>", "<ET><I 610>", "<ET><W 611>", "<ET><E 612>"}
  T55 = typedef "eventvkey.ctl" = enum16{"ASCII", "Enter", "Return", "Shift", "Ctrl", "Alt", "Cmd", "Opt", "Caps", "NumLock", "Clear", "Break", "Up", "Down", "Left", "Right", "Insert", "Delete", "Home", "End", "PageUp", "PageDown", "Escape", "Help", "Pause", "ScrollLock", "F1", "F2", "F3", "F4", "F5", "F6", "F7", "F8", "F9", "F10", "F11", "F12", "F13", "F14", "F15", "F16", "F17", "F18", "F19", "F20", "F21", "F22", "F23", "F24", "Play", "VolumeUp", "VolumeDown", "Mute", "Two Byte Char"}
  T56 = typedef "DB - Master Data Material Enum.ctl" = enum16{"INSERT [MasterData].[Material]", "UPDATE [MasterData].[Material]", "SELECT [MaterialNo]", "SELECT [ShortDescription]", "SELECT [MaterialRev]", "SELECT [Description], [ImageFile]", "SELECT [Description] (Long)"}
  T57 = typedef "DB - Master Data Procedure Enum.ctl" = enum16{"INSERT [MasterData].[Procedure]", "INSERT [MasterData][ProcedureItem]", "SELECT [ProcedureNo]", "SELECT [ProcedureRev]", "SELECT [MasterData].[ProcedureItem]"}
  T58 = typedef "LVSelectionTypeDef.ctl" = cluster{"Selection Start":u32, "Selection End":u32}
  T59 = typedef "NI_LVConfig.lvlib/Config Data RefNum.ctl" = refnum<k1>
  T60 = cluster{"[TransactionNo]":string, "[TransactionRunNo]":string}
  T61 = cluster{"Transaction No":string, "TransactionRunNo":string}
  T62 = typedef "DB - [TransactionResult] Enum.ctl" = enum16{"[StartRecordTime]", "[StartRecordTemp]", "[MaxRecordedTemp]", "[MaxRecordedTempTime]", "[MinRecordedTemp]", "[MinRecordedTempTime]", "[EndRecordTemp]", "[EndRecordTime]", "[RecordedMinutes]", "[StartHoldTime]", "[StartHoldTemp]", "[HoldTimeMaxTemp]", "[HoldTimeMaxTempTime]", "[HoldTimeMinTemp]", "[HoldTimeMinTempTime]", "[EndHoldTime]", "[EndHoldTemp]", "[HoldDurationMinutes]", "[TempDiffDuringHold]", "[UnitOfTemperature]", "[PerformedBy]", "[PerformedOn]", "[IsTempWithinTol]", "[IsTimeWithinTol]", "[HoldTimePercentage]", "[ProcessStatus]", "[OverallStatus]", "[SequenceStatus]", "[Parameter1]", "[Parameter2]", "[Parameter3]", "[Parameter4]", "[Parameter5]", "[Parameter6]", "[Parameter7]", "[Parameter8]", "[Parameter9]", "[Parameter10]", "[Parameter11]", "[Parameter12]", "[Result]", "[RawDataFile]", "[RawDataFilePath]", "[RawDataFileName]", "[OutputSetId]", "[SavedBy]", "[SavedOn]", "[Inactive]"}
  T63 = typedef "DB - [Execute].[ActiveProcess] Enum.ctl" = enum16{"[IsActive]", "[TransactionNo]", "[TransactionRunNo]", "[SequenceStatus]", "[StartRecordTime]", "[EndRecordTime]", "[StartHoldTime]", "[EndHoldTime]", "[Message1]", "[Message2]", "[HoldTimeRemaining]", "[HoldTimePercentage]", "[HoldProgressColor]", "[OrderNumbers]", "[CurrentTemp]", "[UnitOfTemperature]", "[IsAppClientLive]", "[RawDataFile]", "[RecordedMinutes]", "[FurnaceControlStatus]", "[FurnaceControlColor]", "[ControllerStatus]", "[ControllerColor]", "[IsControllerOnline]", "[ProcessColor]", "[OverallColor]", "[LastUpdatedOn]", "[LastUpdatedCmsTime]", "[Inactive]"}
  T64 = typedef "LVPoint32TypeDef.ctl" = cluster{"Horizontal":i32, "Vertical":i32}
  T65 = cluster{"TransactionNo":string, "TransactionRunNo":string}
  T66 = typedef "NI_Database_API.lvlib/Conn ObjectReference.ctl" = refnum<k1>
  T67 = cluster{"TransactionNo":string, "Not Needed for [TransactionRunNo]":string}
  T68 = cluster{"Reports":path, "MasterData\\JPG":path, "String":path, "appended path":path, "Raw Data File (Report Tab)":path, "Temp_Host":path}
  T69 = cluster{"[0]":bool, "[1]":bool, "[2]":bool, "[3]":bool, "[4]":bool, "[5]":bool}
  T70 = cluster{"Value[0]":bool, "Value[1]":bool, "Value[2]":bool, "Value[3]":bool, "Value[4]":bool, "Value[5]":bool}
  T71 = cluster{"Numeric Control":i32, "Numeric Control":i32}
  T72 = typedef "DB - [Config].[Parameters].[ParameterId] Values.ctl" = enum16{"AllowWpsEdit", "ChartSeparation", "DataLogInterval", "DateFormat", "EnableCmsUpdate", "PermittedTempDiff", "PermittedTimeDiff", "StartStopMarker", "DisplayRefChart", "EnableAmsUpdate"}
  T73 = typedef "Key Enum.ctl" = enum16{"String", "Boolean", "NA"}
  T74 = enum16{"INSERT INTO [Execute].[ActiveProcess]", "UPDATE [Execute].[ActiveProcess]", "SELECT [Execute].[ActiveProcess]", "UPDATE FILESTREAM", "SELECT FILESTREAM"}
  T75 = typedef "DB - [Config].[GeneralSetting].[SystemId] Values.ctl" = enum16{"GenericSystemId", "ScreenLockTimer", "TimeSyncSchedule", "TimeSyncTolerance", "TransactStartNo"}
  T76 = cluster{"ProgramNumber":i16, "CurProg":i16, "CurSeg":i16, "ProgStatus":i16, "ProgTimeLeft (min)":dbl, "PVIn (degC)":dbl, "SPIn (NA)":dbl, "SegTimeLeft (min)":dbl}
  T77 = cluster{"Transaction No (Execute)":string, "TransactionRunNo (Execute)":string}
  T78 = cluster{"Start Holding Time & Date":string, "End Holding Time & Date":string, "Start Holding Temperature":string, "End Holding Temperature":string}
diagram:
  w12 = i16 -1  # Segment.Type (unknown)
  w13 = ET3500_Program_Status."Wait For RUN"  # ET3500 Program Status
  w15 = 0  # Sample/ch Count
  w1 = Enum_-_SRTRS_State."QUIT"  # StateMachine for Main Process
  w22 = 20  # Shows Last 20 Events
  w25 = Enum_-_SRTRS_State."READY TO START"  # StateMachine for Main Process
  # "CleanUP"
  n1 = control-ref of="This VI"() -> (w10:refnum<vi>)
  n2 = invoke class="VI" method="Default Vals.Reinit All"(reference=w10) -> (reference out=w9:refnum<vi>, error out=w14:errorcluster)  [unwired: 2 in, 1 out]
  n3 = flat-sequence {
    tunnel: [errorcluster {"status"=FALSE, "code"=0, "source"=""} ("error out")] -> w24
    tunnel: [w73] -> w20
    tunnel: [w245] -> w2
    tunnel: w14 -> [_]
    tunnel: w9 -> [w168]
    frame #0 {
      w122 = "" ("Extra WPS")
      w150 = string[] ["Date and Time", "Transaction No.", "Run No.", "Order No.", "No. of\nOrders", "Report \nRun No.", "Layout ID"]  # 2015-01-12 17:55 Column Header Strings[]
      w154 = string[] ["Name", "Model", "Serial No.", "Last Cal. Date", "Next Cal. Due Date", "Equipment ID", "Notice Period", "Cal. Required"]  # 2015-01-01 11:16 ColHdr[]
      w121 = 4 ("dimension size")
      w135 = u32 6 ("Number of Rows")
      w173 = T34 {"Row"=0, "Column"=0} ("Top Left Visible Cell")
      w199 = string[] ["Sequence Number", "Ramp Rate", "Target Temperature", "Hold Time"] ("Column Header Strings[]")
      w202 = T35 [enum."Page Enabled", enum."Page Enabled", enum."Page Enabled", enum."Page Enabled", enum."Page Enabled"] items=["Page Enabled", "Page Disabled", "Page Disabled & Grayed"]
      w228 = 4 ("dimension size")
      w232 = string[] ["No.", "Order No.", "Oper. No.", "Qty.", "NCR No.", "Customer Name", "Project", "Sales Order", "Item No.", "Material", "Material Description", "Revision", "Serial No.", "TC1", "TC2", "TC3", "TC4", "TC5", "TC6", "TC01Plot", "TC02Plot", "TC03Plot", "TC04Plot", "TC05Plot", "TC06Plot", "Notes", "User", "Customer No.", "NCR Boolean", "UnitOfQty"]  # 2014-09-06 20:13 Column Header Strings[]
      w134 = 2 ("dimension size")
      # "Must set to en, otherwise looking for Config.Messages in DB UI - Logon \nwill have a problem."
      # "Must Create here because the Q uses this Local Variable.\nThe rest can be created after Logon\nThis also means that on 1st Logon, the Log_Host Path , if changed, will not be used.\nThe Data_Host Path and the rest are OK."
      # "Always True, otherwise will skip Logon Screen"
      # "If it's an exe \neg: ver. 2.0.0.41\nRemove last .41\nbecomes ver. 2.0.0"
      # "Not in use"
      # "Set to File Version 1st, will be updated by DB"
      # "Button Controls are initialised at\nTab Body Value Change"
      # "Equipment ID,  Notice Period not shown"
      # "Need to add extra field for ini File"
      # "Visibility Depends on Login User Config Grp"
      # "Parts Details\ncRIO Module Details\nReport List\nFTP File List"
      # "Cannot Put in stp file\notherwise \\0x may have \nproblems"
      # "Material Filename is hidden in the cluster.\n\nCannot put it here, otherwise extra line in report"
      # "These 3 are referenced in \"Report - Excel.vi\" to get the image file  \"<Material>_<Material Description>_<Revision>.jpg\"\n- Material\n- Material Description \n- Revision"
      # "Not copied to Mapped Folder"
      # "Internal Use"
      # "SRTRS4070 Mapped Folder"
      # "SRTRS4070 Host Folder"
      # "EditPos - Initial (KD?) (0)\n                 Initial Text   (1)\n                 B4 (Return) (2)\n                 Now             (3)\n                 Max Row Count  (4)\n(including Last Blank  Row)"
      # "To keep all controls in Part Details to be either MCListBox\nor Clusters"
      # "These are not shown on Part Details MCListbox"
      # "Excluding Notes which makes it 20.\nNotes Column is hidden."
      # "Index# 19"
      # "NumCols set early on top"
      # "All 4 Tabs are here."
      # "Set 1 empty row each"
      # "Initialization"
      n4 = flat-sequence "SETUP TAB" {
        frame #0 {
          w270 = T30."Disabled and Grayed Out" ("Disabled")
          w271 = ""
          n5 = property on="TransactionRunNo" class="Str"("Visible"=FALSE) -> ()  [unwired: 2 in, 2 out]
          n6 = property on="Transaction Details" class="Bool"("Visible"=FALSE) -> ()  [unwired: 2 in, 2 out]
          n7 = property on="Setup Edit" class="Bool (strict)"("DisabledEnum"=T30."Enabled" ("Disabled"), "Value"=TRUE ("Setup Edit")) -> ()  [unwired: 2 in, 2 out]
          n8 = property on="SAPMaterial Description (Long) Setup Tab" class="Bool"("DisabledEnum"=w270) -> ()  [unwired: 2 in, 2 out]
          n9 = property on="SAPProduction Long Text" class="Bool"("DisabledEnum"=w270) -> ()  [unwired: 2 in, 2 out]
          n10 = property on="Output Set" class="CmbBox (strict)"("Strings[]"=string[] [] ("Strings []")) -> ()  [unwired: 2 in, 2 out]
          n11 = property on="Description" class="Str"("Value"="") -> ()  [unwired: 2 in, 2 out]
          "Transaction No" <- w271
          "User" <- w271
          "TransactionRunNo" <- w271
        }
      }
      n12 = disable-structure shown="Disabled" {
        frame Disabled {
          n13 = control-ref of="Tab Body"() -> (w279:refnum<vi>)
          n14 = call "Tabs - Page Visibility.vi"("TabControl in"=w279) -> ()  [unwired: 10 in, 1 out]
        }
        frame Enabled {
        }
      }
      n15 = case shown="\"Header\", Default" enum16{"Header", "Body", "Debug"}."Header" {
        tunnel: [T32 {"Horizontal"=0, "Vertical"=0} ("Origin") T32 {"Horizontal"=0, "Vertical"=75} ("Origin") T32 {"Horizontal"=0, "Vertical"=200} ("Origin")] -> w236
        frame "Header", Default {
        }
        frame "Body" {
        }
        frame "Debug" {
        }
      }
      n16 = flat-sequence "EXECUTE TAB (xx Controls)" {
        frame #0 {
          w313 = "" ("TransactionRunNo")
          w314 = T36 [{"Color Box"=9868950, "Color Box 2"=9868950}, {"Color Box"=6618880, "Color Box 2"=6618880}, {"Color Box"=4934475, "Color Box 2"=4934475}, {"Color Box"=6618880, "Color Box 2"=6618880}]  # Init
          w322 = T30."Disabled and Grayed Out" ("Disabled")
          w312 = T10 {"Recording Duration"=0.0, "Remaining Hold Time"=0.0, "Current Temp"=0.0, "Key Values Temperature Units"="°C"} ("Key Values")
          w310 = "" ("Transaction No 2")
          # "Initialize"
          n17 = flat-sequence {
            frame #0 {
              w342 = T36 [{"Color Box"=9868950, "Color Box 2"=9868950}, {"Color Box"=6618880, "Color Box 2"=6618880}, {"Color Box"=4934475, "Color Box 2"=4934475}, {"Color Box"=6618880, "Color Box 2"=6618880}]  # Init
              w343 = FALSE ("Value")
              n18 = property on="Variant Allowed (Hold Temp)" class="Bool (strict)"("Colors [4]"=w342, "Value"=w343) -> ()  [unwired: 2 in, 2 out]
              n19 = property on="Variant Allowed (Hold Time)" class="Bool (strict)"("Colors [4]"=w342, "Value"=w343) -> ()  [unwired: 2 in, 2 out]
              "Info." <- T9 {"Ref WPS"="", "Hold. Temp."="", "Info. Temperature Units"="", "Variant Allowed (Hold Temp)"=0.0, "Info. Temperature Units 2"="", "Variant Allowed (Hold Temp)"=FALSE, "Hold. Time (hour:minute)"="", "Variant Allowed (Hold Time)"=30.0, "Variant Allowed (Hold Time)"=FALSE, "WPS"=""} ("Info.")
            }
          }
          n20 = control-ref of="ET3504 Status"() -> (w321:refnum<vi>)
          n21 = global write "Global SRTRS.vi" "[TransactionRunNo]"(w313) -> ()
          n22 = global read "Global SRTRS.vi" "Temperature Units"() -> (w311:string)
          n23 = Bundle By Name(cluster=w312, "Key Values Temperature Units"=w311) -> ()  [unwired: 1 out]
          n24 = global write "Global SRTRS.vi" "[TransactionNo]"(w310) -> ()
          n25 = property class="Str"(reference=w321, "Text.BG Color"=u32 16777216 ("ET3500 Transparent Color")) -> ()  [unwired: 1 in, 2 out]
          n26 = control-ref of="cRIO Status"() -> (w318:refnum<vi>)
          n27 = flat-sequence {
            frame #0 {
              w337 = 0.0 ("% Hold Time Completed")
              n28 = property on="% Hold. Time Completed" class="Slide (strict)"("Scale.Maximum"=100.0 ("Scale.Range:Maximum"), "Scale.Minimum"=0.0 ("Scale.Range:Minimum"), "Fill Color"=u32 16777216 ("Color Box 2"), "Value"=0.0 ("% Hold Time Completed")) -> ()  [unwired: 2 in, 2 out]
              "% Hold. Time Completed" <- w337
              "% Hold. Time Completed (Num)" <- w337
            }
          }
          n29 = property class="Str"(reference=w318, "Text.BG Color"=u32 16777216 ("ET3500 Transparent Color")) -> ()  [unwired: 1 in, 2 out]
          n30 = flat-sequence {
            frame #0 {
              w329 = 12  # 12 Probes Max
              n31 = property on="Chart" class="WFChart (strict)"("History Data"=dynamicdata[] [[{"t0"=timestamp(3471350400 s since 1904-01-01), "dt"=1.0, "Y"=[0.0, 0.0]}]]) -> (error out=w328:errorcluster)  [unwired: 2 in, 1 out]
              n32 = for {
                N: w329 -> [_]
                i -> [w336]
                n33 = property on="Chart" class="WFChart (strict)"("Active Plot"=w336, "Plot.Plot Name"="") -> ()  [unwired: 2 in, 2 out]
              }
              n34 = disable-structure shown="Disabled" {
                disable-tunnel: w328 -> [w330 _]
                frame Disabled {
                  # "1 hour"
                  n35 = Get Date/Time In Seconds() -> (seconds since 1Jan1904=w334:timestamp)
                  n36 = To Double Precision Float(number=w334) -> (double precision float=w333:dbl)
                  n37 = Add(x=w333, y=3600.0) -> (x+y=w331:dbl)
                  n38 = property on="Chart" class="WFChart (strict)"(error in=w330, "XScale.Minimum"=w333, "XScale.Maximum"=w331) -> ()  [unwired: 1 in, 2 out]
                }
                frame Enabled {
                }
              }
            }
          }
          n39 = property on="Recipe Start" class="Bool"("DisabledEnum"=w322) -> ()  [unwired: 2 in, 2 out]
          n40 = property on="Recipe Stop" class="Bool"("DisabledEnum"=w322) -> ()  [unwired: 2 in, 2 out]
          n41 = property on="Hold Time Completed" class="Bool (strict)"("Colors [4]"=w314) -> ()  [unwired: 2 in, 2 out]
          n42 = property on="Overall Status" class="Bool (strict)"("Colors [4]"=w314) -> ()  [unwired: 2 in, 2 out]
          n43 = property on="Process Completed" class="Bool (strict)"("Colors [4]"=w314) -> ()  [unwired: 2 in, 2 out]
          "Transaction No (Execute)" <- w310
          "Key Values" <- w312
          "ET3504 Status" <- "Offline." ("ET3500 Program Status")
          "cRIO Status" <- "Offline." ("cRIO Status")
          "Process Completed" <- FALSE ("Overall Status")
          "No. of Items" <- 0 ("No. of Items")
          "Sequence Status" <- "" ("Sequence Status")
          "Overall Status" <- FALSE ("Overall Status")
          "Hold Time Completed" <- FALSE ("Hold Time Completed")
          "TransactionRunNo (Execute)" <- w313
        }
      }
      n44 = Current VI's Path() -> (path=→"Current VI's path":path)
      n45 = call <vilib>:"Application Directory.vi"() -> ("Application Directory"=w81:path)
      "Application Directory" <- w81
      n46 = property class="VI"(reference=w168) -> (reference out=w166:refnum<vi>, "Panel"=w167:refnum<vi>)  [unwired: 1 in, 1 out]
      n47 = global write "Global SRTRS.vi" "Main Application Directory"(w81) -> ()
      n48 = property on="Pane" class="Pane"("Origin"=w236) -> ()  [unwired: 2 in, 2 out]
      n49 = control-ref of="MCListBox FHS Setup Remove Button"() -> (w170:refnum<vi>)
      n50 = control-ref of="MCListBox FHS Setup Add Button"() -> (w169:refnum<vi>)
      n51 = property class="Pnl"(reference=w167) -> ("Panes[]"=w165:refnum<vi>[])  [unwired: 1 in, 2 out]
      n52 = control-ref of="No."() -> (w93:refnum<vi>)
      n53 = control-ref of="Tab Setup"() -> (w103:refnum<vi>)
      n54 = Index Array(array=w165) -> (element=w164:refnum<vi>)  [unwired: 1 in]
      n55 = property class="Bool"(reference=w170, "Visible"="Edit WPS in Setup") -> ()  [unwired: 1 in, 2 out]
      n56 = property class="Bool"(reference=w169, "Visible"="Edit WPS in Setup") -> ()  [unwired: 1 in, 2 out]
      n57 = property class="VI"(reference=w166) -> ("Metric.CodeSize"=w184:u32)  [unwired: 1 in, 2 out]
      "Metrics:Code Size" <- w184
      n58 = call "Setup Tab - Enable-Disable.vi"("No."=w93, "[SRTRS][Config][ParameterSettings] - [userEditableProcedure]"="Edit WPS in Setup", "Disabled"=T30."Enabled", "Tab Setup"=w103) -> ()  [unwired: 8 in]
      n59 = property on="Tab Body" class="TabCtl (strict)"() -> ("Pages"=w203:refnum<vi>[])  [unwired: 2 in, 2 out]
      n60 = local write "Equipment Details"(-1 ("Temperature Module Calibration")) -> ()
      n61 = global write "Global SRTRS.vi" "Logon"(T21 {"PlantID"="", "SystemID"="", "UserID"="", "DomainID"="", "LanguageID"="en", "StationID"=""} ("Logon")) -> ()
      n62 = for {
        tunnel: w203 -> [w354] mode=indexing
        tunnel: w202 -> [w353] mode=indexing
        n63 = property class="Page"(reference=w354, "PageEnb"=w353) -> ()  [unwired: 1 in, 2 out]
      }
      n64 = Format Into String(format string="%d.", initial string="Code Size = ", w184) -> (resulting string=w181:string)  [unwired: 1 in, 1 out]
      n65 = disable-structure shown="Disabled" {
        frame Disabled {
          n66 = property on="Tab Setup" class="TabCtl (strict)"() -> ("Pages"=w348:refnum<vi>[])  [unwired: 2 in, 2 out]
          n67 = property on="Master Data Tab" class="TabCtl (strict)"() -> ("Pages"=w347:refnum<vi>[])  [unwired: 2 in, 2 out]
          n68 = Build Array (concatenate)(w348, w347) -> (w346:refnum<vi>[])
          n69 = for {
            tunnel: w346 -> [w350] mode=indexing
            tunnel: [w349] -> w345 mode=concatenating
            n70 = property class="Page"(reference=w350) -> ("ControlsOnPage"=w349:refnum<vi>[])  [unwired: 1 in, 2 out]
          }
          n71 = for {
            tunnel: w345 -> [w352] mode=indexing
            # "Show Labels for Debugging"
            # "Show/Hide All Labels"
            n72 = property class="Ctl"(reference=w352, "Label.Visible"=FALSE) -> ()  [unwired: 1 in, 2 out]
          }
        }
        frame Enabled {
        }
      }
      n73 = control-ref of="MCListBox FHS Setup"() -> (w114:refnum<vi>)
      n74 = control-ref of="MCListBox AWPS"() -> (w108:refnum<vi>)
      n75 = control-ref of="Part Details"() -> (w106:refnum<vi>)
      n76 = control-ref of="Equipment Details"() -> (w97:refnum<vi>)
      n77 = control-ref of="Tab Setup"() -> ()  [unwired: 1 out]
